vi "GLIMPSE Sequence Read.vi"() -> ()   [LabVIEW 2011]
doc: "Takes a collection of frames stored on the disk in one of several formats and stores them as a Glimpse sequence file."
uses:
  GLIMPSE Globals.vi
panel:
  in  "Number of acquisition files":i32=10
  in  "Used for TIFFs and stacked TIFFs only.\nFor stacked TIFFs, set to zero to \nread times from .MAT file.":dbl caption="Milliseconds per frame" format="%.2f"
  out "Acquiring?":bool
  in  "New":bool
  in  "Over-write":bool=TRUE
  in  "Save into new directory:":path=path "d:/1.glimpse"
  in  "Over-write exisitng:":path=path "d:/1.glimpse"
  in  "Go?":bool
  in  "stop":bool
  in  "File Format Options":i32(listbox)
  # "Make any changes required, then press"
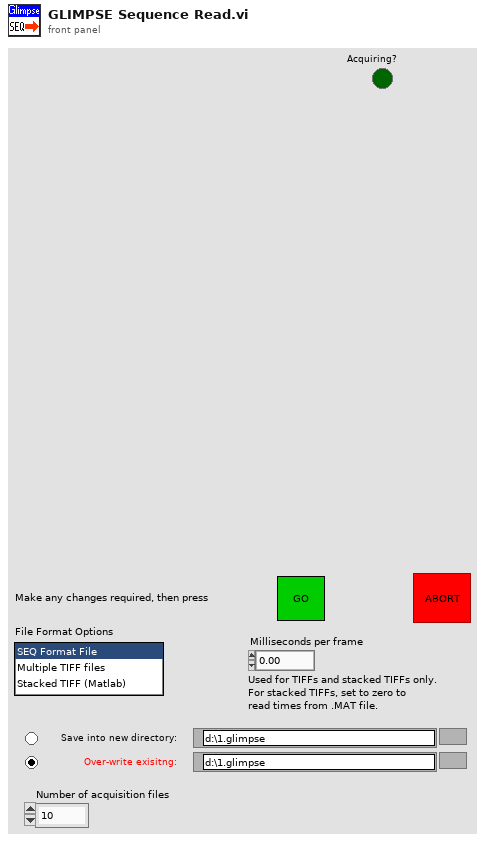
[diagram p1: front panel]
types:
  T1 = typedef "Sequence files handle.ctt" = cluster{"Sequence files directory path":path, "Sequence files refnum array":refnum<file>[]}
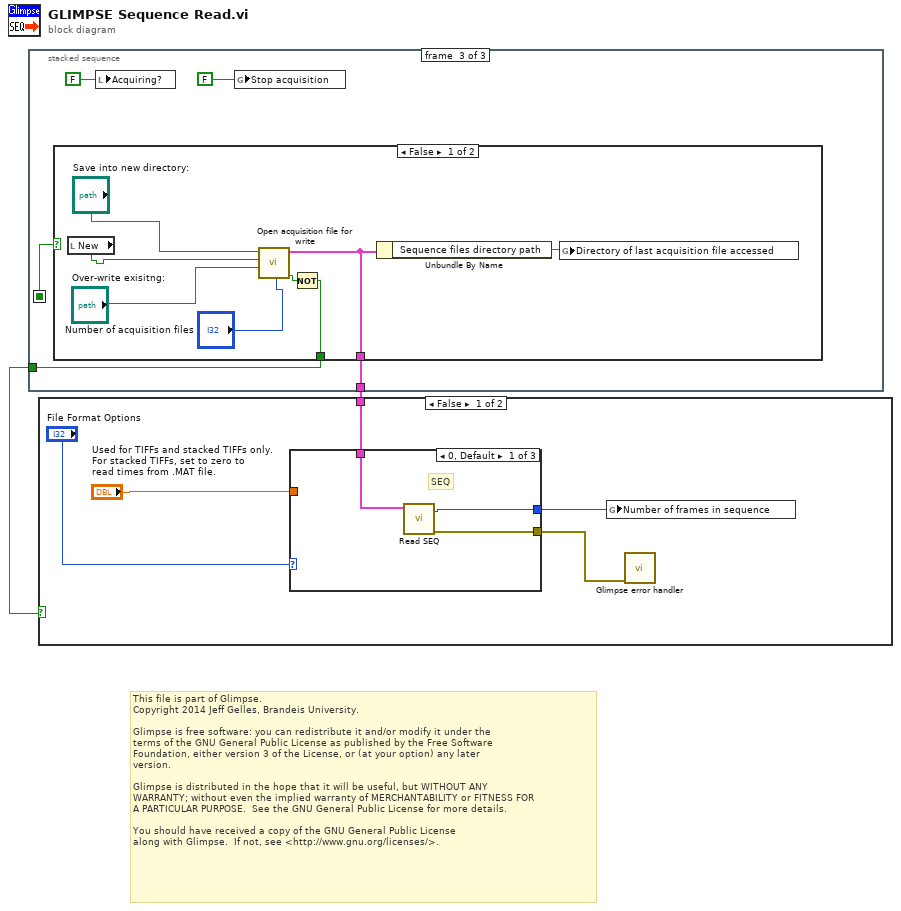
[diagram p0: block diagram]
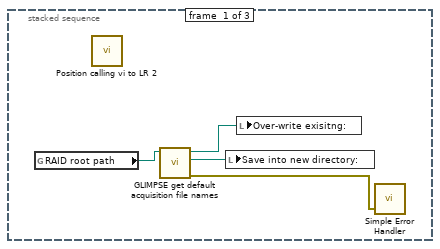
[diagram p2: hidden frame]
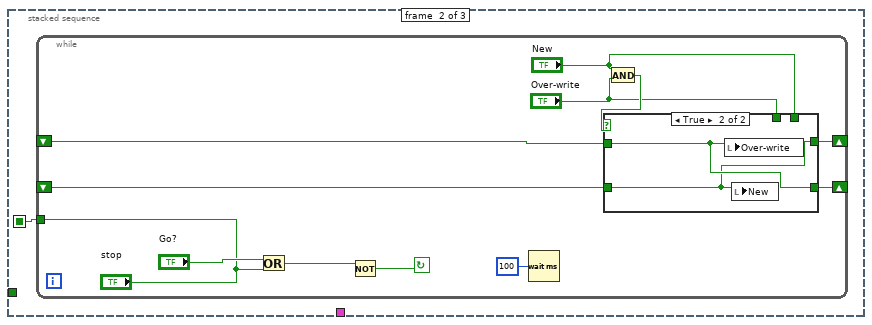
[diagram p3: hidden frame]
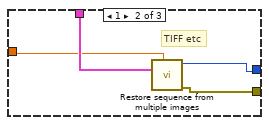
[diagram p6: hidden frame]
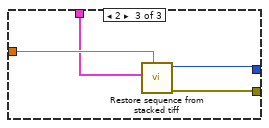
[diagram p7: hidden frame]
diagram:
  # "This file is part of Glimpse. \nCopyright 2014 Jeff Gelles, Brandeis University.    \n\nGlimpse is free software: you can redistribute it and/or modify it under the \nterms of the GNU General Public License as published by the Free Software \nFoundation, either version 3 of the License, or (at your option) any later \nversion.\n\nGlimpse is distributed in the hope that it will be useful, but WITHOUT ANY \nWARRANTY; without even the implied warranty of MERCHANTABILITY or FITNESS FOR \nA PARTICULAR PURPOSE.  See the GNU General Public License for more details.\n\nYou should have received a copy of the GNU General Public License\nalong with Glimpse.  If not, see <http://www.gnu.org/licenses/>."
  n1 = stacked-sequence {
    seq-local: [_ w7 _] -> [_ _ w24]
    tunnel: [_ _ w26] -> w2
    tunnel: [_ _ w25] -> w1
    frame #0 {
      n2 = global read "GLIMPSE Globals.vi" "RAID root path"() -> (w4:path)
      n3 = call "Position calling vi to LR 2.vi"() -> ()  [unwired: 2 in, 4 out]
      n4 = call "GLIMPSE get default acquisition file names.vi"("RAID root path"=w4) -> ("error out"=w3:errorcluster, "next directory path"=w5:path, "last directory path"=w6:path)  [unwired: 1 in, 5 out]
      n5 = local write "Save into new directory:"(w5) -> ()
      n6 = local write "Over-write exisitng:"(w6) -> ()
      n7 = call <vilib>:"Simple Error Handler.vi"("error in (no error)"=w3) -> ()  [unwired: 1 in, 8 out]
    }
    frame #1 {
      n8 = while {
        tunnel: ["stop"] -> w7
        shift-right: [w9] -> _
        shift-left: _ -> [w11]
        shift-right: [w8] -> _
        shift-left: _ -> [w10]
        stop <- w18 continue-if-true
        n9 = Or(x="Go?", y="stop") -> (x .or. y?=w16:bool)
        n10 = Not(x=w16) -> (.not. x?=w18:bool)
        n11 = Wait (ms)(milliseconds to wait=u32 100) -> ()  [unwired: 1 out]
        n12 = And(x="New", y="Over-write") -> (x .and. y?=w14:bool)
        n13 = case shown="True" w14 {
          tunnel: [w21 w22] -> w9
          tunnel: "New" -> [w21 _]
          tunnel: "Over-write" -> [w20 _]
          tunnel: [w20 w23] -> w8
          tunnel: w11 -> [_ w23]
          tunnel: w10 -> [_ w22]
          frame False {
          }
          frame True {
            n14 = local write "Over-write"(w23) -> ()
            n15 = local write "New"(w22) -> ()
          }
        }
      }
    }
    frame #2 {
      n16 = case shown="False" w24 {
        selector: w24 -> [_ w37]
        tunnel: [w32 w37] -> w26
        tunnel: [w30 _] -> w25
        frame False {
          n17 = local read "New"() -> (w34:bool)
          n18 = call "Open acquisition file for write.vi"("Number of acquisition files"="Number of acquisition files", "Existing directory to over-write"="Over-write exisitng:", "Use new?"=w34, "New directory to create"="Save into new directory:") -> ("OK?"=w33:bool, "Sequence files handle"=w30:T1)  [unwired: 5 out]
          n19 = Not(x=w33) -> (.not. x?=w32:bool)
          n20 = Unbundle By Name(w30) -> ("Sequence files directory path"=w31:path)
          n21 = global write "GLIMPSE Globals.vi" "Directory of last acquisition file accessed"(w31) -> ()
        }
        frame True {
        }
      }
      n22 = local write "Acquiring?"(FALSE ("stop")) -> ()
      n23 = global write "GLIMPSE Globals.vi" "Stop acquisition"(FALSE ("Stop acquisition")) -> ()
    }
  }
  n24 = case shown="False" w2 {
    tunnel: w1 -> [w41 _]
    frame False {
      n25 = case shown="0, Default" "File Format Options" {
        tunnel: w41 -> [w45 w49 w50]
        tunnel: [w44 w48 w53] -> w40
        tunnel: "Used for TIFFs and stacked TIFFs only.\nFor stacked TIFFs, set to zero to \nread times from .MAT file." -> [_ w47 w51]
        tunnel: [w43 w46 w52] -> w38
        frame 0, Default {
          # "SEQ"
          n26 = call "Read SEQ.vi"("Sequence files handle"=w45) -> ("error out"=w43:errorcluster, "# of Frames"=w44:i16)  [unwired: 1 in, 7 out]
        }
        frame 1 {
          # "TIFF etc"
          n27 = call "Restore sequence from multiple images.vi"("Milliseconds per frame"=w47, "Sequence files handle"=w49) -> ("error out"=w46:errorcluster, "Last frame number written out"=w48:u32)  [unwired: 2 in, 5 out]
        }
        frame 2 {
          n28 = call "Restore sequence from stacked tiff.vi"("Milliseconds per frame"=w51, "Sequence files handle"=w50) -> ("error out"=w52:errorcluster, "Last frame number written out"=w53:u32)  [unwired: 2 in, 5 out]
        }
      }
      n29 = global write "GLIMPSE Globals.vi" "Number of frames in sequence"(w40) -> ()
      n30 = call "Glimpse error handler.vi"("error in"=w38) -> ()  [unwired: 1 in, 6 out]
    }
    frame True {
    }
  }
